vi "Driver - DTACQ - Download Captured Data (Multiplexed - Signed 16 Bit).vi"(8 "error in":errorcluster, 10 "Samples":i32, 11 "DTACQ Connection Data In":T1={"Description"="", "Address"="", "Port"=0, "timeout (ms)"=5000, "Termination Character"="\n", "TCP Connection Reference"=refnum, "Open Connection"=FALSE}) -> (0 "error out":errorcluster, 1 "Timed Out":bool=TRUE, 2 "(Signed) 16 Bit Array":i16[](array[numeric]), 3 "DTACQ Connection Data Out":T1={"Description"="", "Address"="", "Port"=0, "timeout (ms)"=5000, "Termination Character"="\n", "TCP Connection Reference"=refnum, "Open Connection"=FALSE})   [LabVIEW 2017, in "Communications Library.lvlib"]
doc: "Downloads binary data from the DTACQ device. \n\nData is read as a stream of bytes, and is then converted to 1D array of signed 16 bit numbers.\nThe stream of bytes is assumed to be in little-endian format."
uses:
  Communications Library.lvlib
  Typedefs/DTACQ Connection Data--Cluster.ctl
  Debug - Lower Level - Logging Tool.vi
  Error 5102 - DTACQ unit replied with an error--const.vi
  <vilib>/Utility/error.llb/Error Cluster From Error Code.vi
  Debug - TCP - Create Descriptive String.vi
  Debug - TCP - Write to Log File.vi
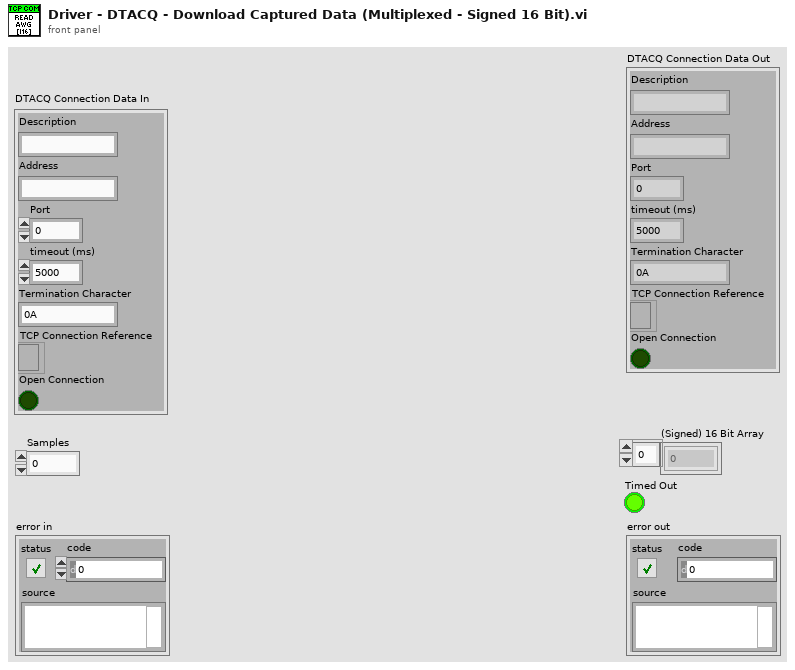
[diagram p1: front panel]
types:
  T1 = typedef "Communications Library.lvlib/DTACQ Connection Data--Cluster.ctl" = cluster{"Description":string, "Address":string, "Port":u16, "timeout (ms)":i32, "Termination Character":string, "TCP Connection Reference":refnum<k5>, "Open Connection":bool}
  T2 = enum16{"Little-Endian (LSBF)", "Big-Endian (MSBF)"}
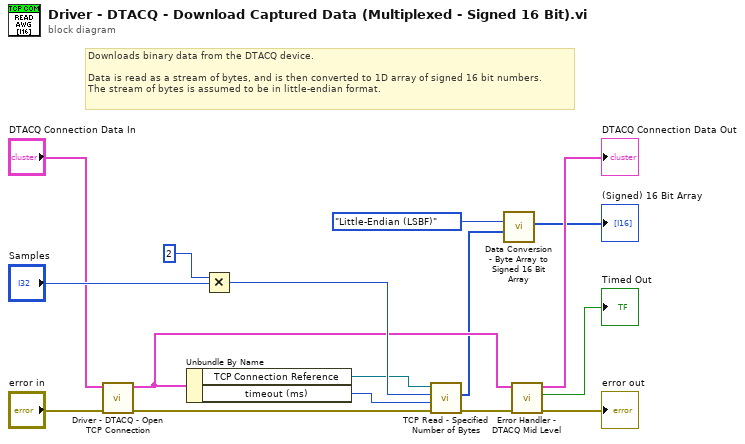
[diagram p0: block diagram]
diagram:
  # "Downloads binary data from the DTACQ device.  \n\nData is read as a stream of bytes, and is then converted to 1D array of signed 16 bit numbers.\nThe stream of bytes is assumed to be in little-endian format."
  n1 = call "Driver - DTACQ - Open TCP Connection.vi"("error in"="error in", "DTACQ Connection Data In"="DTACQ Connection Data In") -> ("error out"=w9:errorcluster, "DTACQ Connection Data Out"=w5:T1)  [unwired: 8 in]
  n2 = Unbundle By Name(w5) -> ("TCP Connection Reference"=w12:refnum<k5>, "timeout (ms)"=w13:i32)
  n3 = Multiply(x=u16 2, y="Samples") -> (x*y=w14:i32)
  n4 = call "TCP Read - Specified Number of Bytes.vi"("error in"=w9, "Timeout ms (default 50ms)"=w13, "Bytes to Read"=w14, "TCP Network Connection in"=w12) -> ("error out"=w8:errorcluster, "Unsigned Byte Array"=w2:u8[])  [unwired: 5 in, 1 out]
  n5 = call "Data Conversion - Byte Array to Signed 16 Bit Array.vi"("Unsigned Byte Array"=w2, "Byte Order"=T2."Little-Endian (LSBF)") -> ("(Signed) 16 Bit Array"=→"(Signed) 16 Bit Array":i16[])  [unwired: 9 in]
  n6 = call "Error Handler - DTACQ Mid Level.vi"("error in"=w8, "DTACQ Connection Data In"=w5) -> ("error out"=→"error out":errorcluster, "Timed Out"=→"Timed Out":bool, "DTACQ Connection Data Out"=→"DTACQ Connection Data Out":T1)  [unwired: 7 in]
